vi "TeilA.vi"() -> ()   [LabVIEW 2010]
uses:
  <vilib>/Utility/file.llb/Write To Spreadsheet File (DBL).vi
  <vilib>/Analysis/NI_AALBase.lvlib
panel:
  out "Tank":dbl(slide) scale=0.0..100.0
  out "Progress":u8(slide) scale=0.0..100.0
  out "Waveform Chart Phasen":dbl(graph)
  out "Waveform Chart Amplituden":dbl(graph)
  out "Amplitude vs Phase":cluster{dbl[], dbl[]}(graph)
  out "Freq vs PhasError":cluster{dbl[], dbl[]}(graph)
  out "Freq vs PhasMean":cluster{dbl[], dbl[]}(graph)
  out "Freq vs AmpError":cluster{dbl[], dbl[]}(graph)
  out "Freq vs AmpMean":cluster{dbl[], dbl[]}(graph)
  out "Inner Loop\nIndicator":i32
  out "Outer Loop\nIndicator":i32
  in  "mode (0) 2":i16
  in  "address Freq":string="19"
  out "Frequenz in Hz":dbl=200.0 format="%.2f"
  in  "Wait/s":dbl=1.0 format="%.2f"
  in  "Step":dbl=1.0 format="%.2f"
  out "current frequency value":string
  out "error out 2":errorcluster
  in  "error in (no error) 2":errorcluster
  in  "Stop":dbl=205.0 format="%.2f"
  in  "Freq Start":dbl=200.0 format="%.2f"
  out "Phasen Error":dbl
  out "Phasen Mean":dbl
  out "Amplituden Error":dbl
  out "Amplituden Mean":dbl
  out "Phasen":dbl[](array[numeric])
  out "Amplituden":dbl[](array[numeric])
  out "data X":dbl format="%#_6e"
  out "data Y":dbl
  in  "mode (0)":i16
  in  "address LockIn":string="7"
  out "Counter":dbl[](array[numeric])
  in  "Path":path
  in  "Start":dbl format="%.2f"
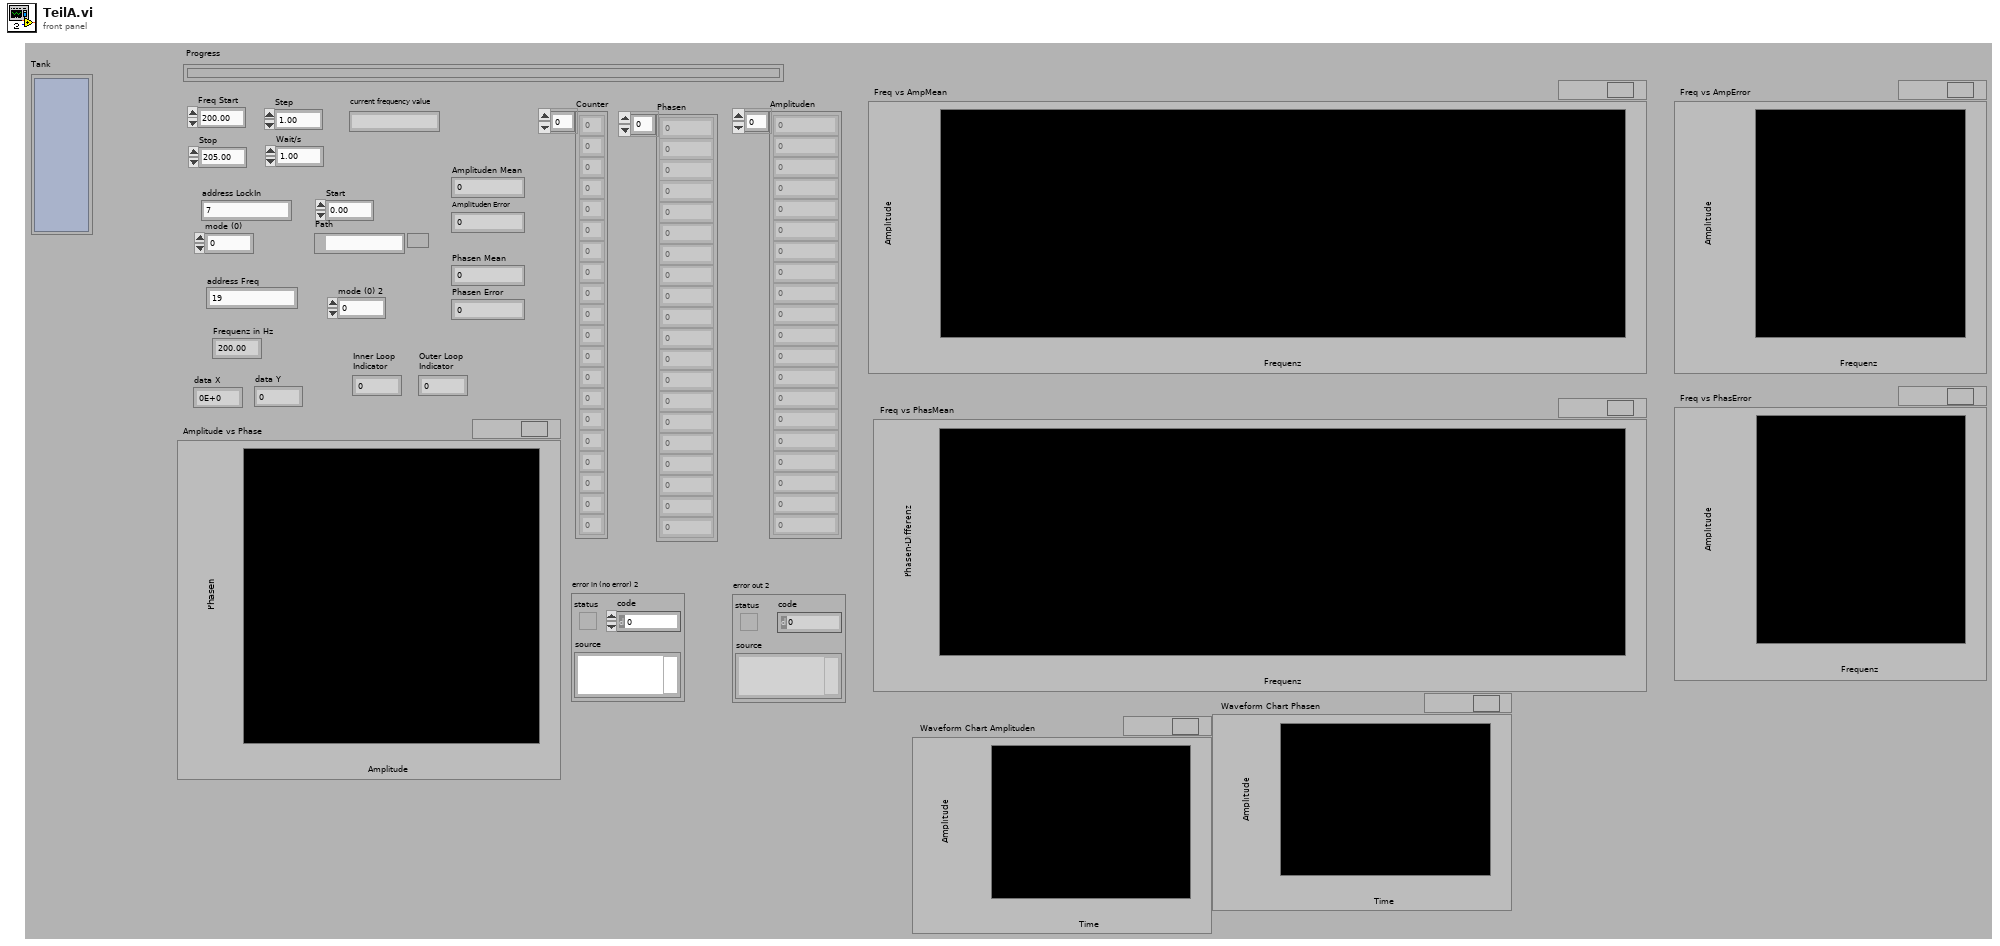
[diagram p1: front panel]
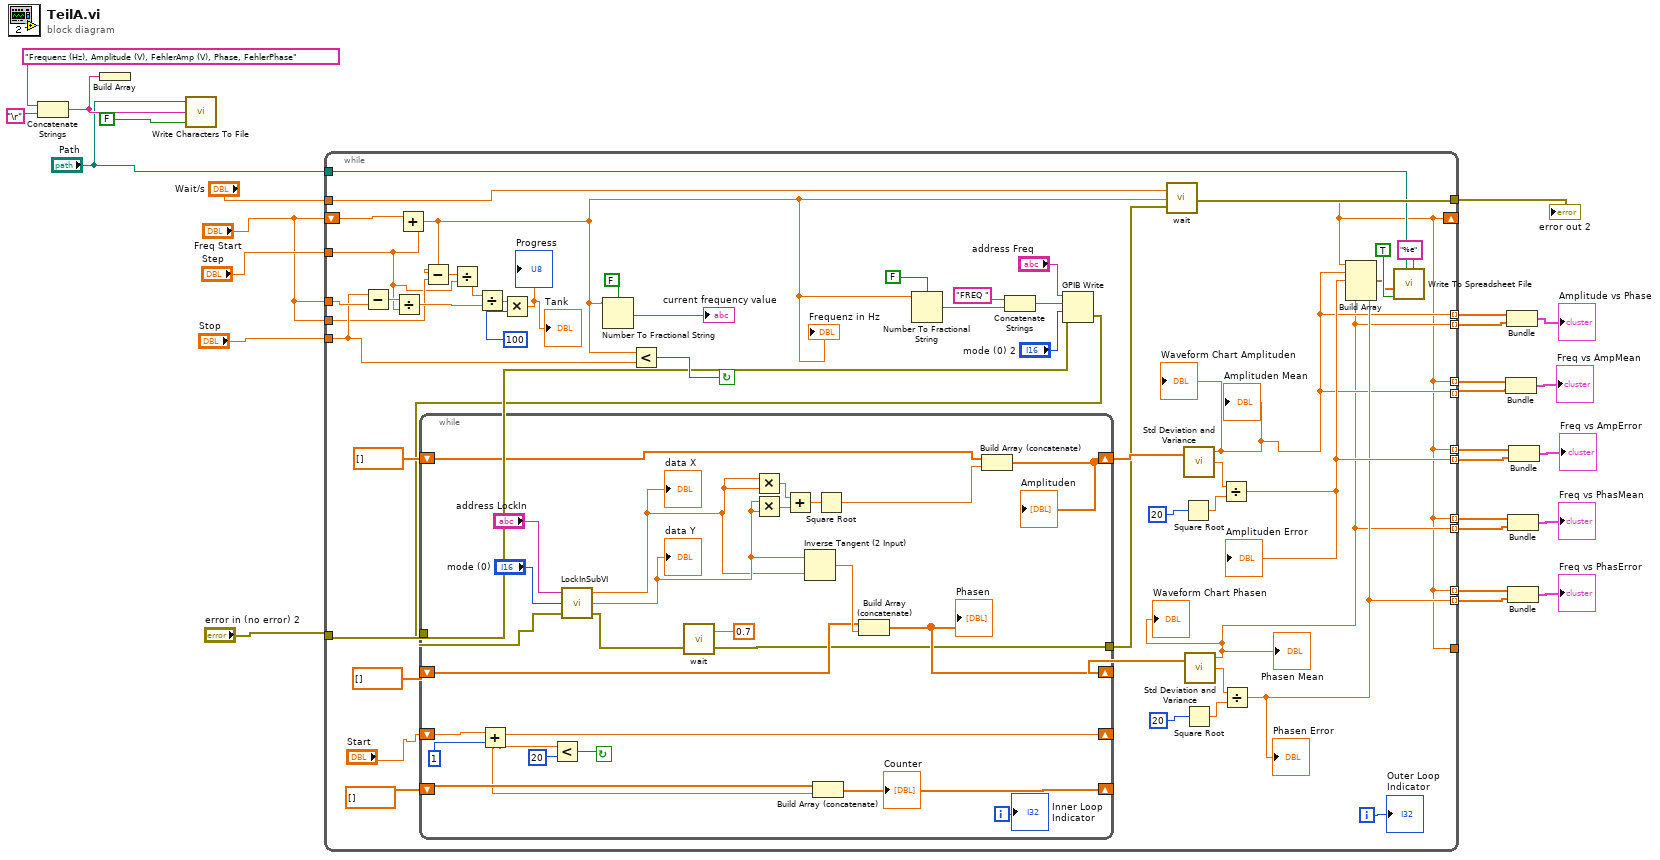
[diagram p0: block diagram]
diagram:
  n1 = Concatenate Strings("Frequenz (Hz), Amplitude (V), FehlerAmp (V), Phase, FehlerPhase", "\r") -> (w18:string)
  n2 = Build Array(w18) -> ()  [unwired: 1 out]
  n3 = call <vilib>:"Write Characters To File.vi"("append to file? (new file:F)"=FALSE, "character string"=w18, "file path (dialog if empty)"="Path") -> ()  [unwired: 2 in, 1 out]
  n4 = while {
    tunnel: "error in (no error) 2" -> [w47]
    tunnel: [w73] -> w26
    shift-right: [w32] -> _
    shift-left: "Freq Start" -> [w36]
    tunnel: "Step" -> [w28]
    tunnel: "Stop" -> [w34]
    tunnel: "Wait/s" -> [w72]
    tunnel: "Path" -> [w55]
    tunnel: [w32] -> _
    tunnel: [w32] -> w16 mode=indexing
    tunnel: [w42] -> w15 mode=indexing
    tunnel: [w32] -> w12 mode=indexing
    tunnel: [w44] -> w11 mode=indexing
    tunnel: [w32] -> w9 mode=indexing
    tunnel: [w41] -> w8 mode=indexing
    tunnel: [w32] -> w6 mode=indexing
    tunnel: [w43] -> w5 mode=indexing
    tunnel: [w42] -> w3 mode=indexing
    tunnel: [w41] -> w2 mode=indexing
    tunnel: "Freq Start" -> [w35]
    tunnel: "Freq Start" -> [w31]
    i -> [w40]
    stop <- w74 continue-if-true
    n5 = Subtract(x=w34, y=w35) -> (x-y=w37:dbl)
    n6 = Divide(x=w37, y=w28) -> (x/y=w33:dbl)
    n7 = Add(x=w36, y=w28) -> (x+y=w32:dbl)
    "Frequenz in Hz" <- w32
    n8 = Subtract(x=w32, y=w31) -> (x-y=w29:dbl)
    n9 = Divide(x=w29, y=w28) -> (x/y=w30:dbl)
    n10 = Divide(x=w30, y=w33) -> (x/y=w38:dbl)
    n11 = Multiply(x=w38, y=100) -> (x*y=→"Progress" →"Tank":dbl)
    n12 = Number To Fractional String(use system decimal point (T)=FALSE, number=w32) -> (F-format string=→"current frequency value":string)  [unwired: 2 in]
    n13 = Less?(x=w32, y=w34) -> (x < y?=w74:bool)
    n14 = Number To Fractional String(use system decimal point (T)=FALSE, number=w32) -> (F-format string=w51:string)  [unwired: 2 in]
    n15 = Concatenate Strings("FREQ ", w51) -> (w50:string)
    n16 = GPIB Write(0:"address Freq", 1:w50, 2:"mode (0) 2", 3:w47) -> (6:w46:errorcluster)  [unwired: 1 in, 1 out]
    n17 = while {
      tunnel: w46 -> [w83]
      shift-right: [w78] -> _
      shift-left: "Start" -> [w98]
      shift-right: [w79] -> _
      shift-left: dbl[] [] -> [w80]
      shift-right: [w88] -> w60
      shift-left: dbl[] [] -> [w89]
      shift-right: [w85] -> w67
      shift-left: dbl[] [] -> [w86]
      tunnel: [w77] -> w48
      i -> [w75]
      stop <- w81 continue-if-true
      n18 = Add(x=w98, y=1) -> (x+y=w78:dbl)
      n19 = Less?(x=w78, y=20) -> (x < y?=w81:bool)
      n20 = call "LockInSubVI.vi"("error in"=w83, "mode (0)"="mode (0)", "address string"="address LockIn") -> ("error out 2"=w76:errorcluster, "data Y"=w92:dbl, "data X"=w91:dbl)
      "data Y" <- w92
      "data X" <- w91
      n21 = call "wait.vi"("error in"=w76, "Wartezeit in Sek"=0.7) -> ("error out"=w77:errorcluster)  [unwired: 1 in]
      n22 = Multiply(x=w91, y=w91) -> (x*y=w95:dbl)
      n23 = Multiply(x=w92, y=w92) -> (x*y=w94:dbl)
      n24 = Add(x=w95, y=w94) -> (x+y=w93:dbl)
      n25 = Inverse Tangent (2 Input)(1:w91, 2:w92) -> (0:w87:dbl)
      n26 = Build Array (concatenate)(w80, w78) -> (w79:dbl[])
      "Counter" <- w79
      n27 = Square Root(x=w93) -> (sqrt(x)=w90:dbl)
      n28 = Build Array (concatenate)(w86, w87) -> (w85:dbl[])
      "Phasen" <- w85
      n29 = Build Array (concatenate)(w89, w90) -> (w88:dbl[])
      "Amplituden" <- w88
      "Inner Loop\nIndicator" <- w75
    }
    n30 = call "wait.vi"("error in"=w48, "Wartezeit in Sek"=w72) -> ("error out"=w73:errorcluster)  [unwired: 1 in]
    n31 = Square Root(x=20) -> (sqrt(x)=w63:dbl)
    n32 = call <vilib>:"Std Deviation and Variance.vi"("X"=w60) -> ("mean"=w42:dbl, "standard deviation"=w61:dbl)  [unwired: 1 in, 1 out]
    "Amplituden Mean" <- w42
    "Waveform Chart Amplituden" <- w42
    n33 = Square Root(x=20) -> (sqrt(x)=w66:dbl)
    n34 = call <vilib>:"Std Deviation and Variance.vi"("X"=w67) -> ("mean"=w41:dbl, "standard deviation"=w64:dbl)  [unwired: 1 in, 1 out]
    "Phasen Mean" <- w41
    "Waveform Chart Phasen" <- w41
    n35 = Divide(x=w61, y=w63) -> (x/y=w44:dbl)
    "Amplituden Error" <- w44
    n36 = Divide(x=w64, y=w66) -> (x/y=w43:dbl)
    "Phasen Error" <- w43
    n37 = Build Array(w32, w42, w44, w41, w43) -> (w45:dbl[])
    n38 = call-poly <vilib>:"Write To Spreadsheet File.vi"("format (%.3f)"="%e", "append to file? (new file:F)"=TRUE, "1D data"=w45, "file path (dialog if empty)"=w55) -> ()  [unwired: 4 in, 1 out]
    "Outer Loop\nIndicator" <- w40
  }
  "error out 2" <- w26
  n39 = Bundle(w16, w15) -> (→"Freq vs AmpMean":cluster{dbl[], dbl[]})  [unwired: 1 in]
  n40 = Bundle(w3, w2) -> (→"Amplitude vs Phase":cluster{dbl[], dbl[]})  [unwired: 1 in]
  n41 = Bundle(w9, w8) -> (→"Freq vs PhasMean":cluster{dbl[], dbl[]})  [unwired: 1 in]
  n42 = Bundle(w6, w5) -> (→"Freq vs PhasError":cluster{dbl[], dbl[]})  [unwired: 1 in]
  n43 = Bundle(w12, w11) -> (→"Freq vs AmpError":cluster{dbl[], dbl[]})  [unwired: 1 in]
